vi "IMU_Read_STATUS.vi"(8 "error in (no error)":errorcluster caption="Fehler (Eingang, kein Fehler)", 10 "VISA resource name IN":refnum<visa-resource-name>, 11 "MultiWii Data Cluster 2":refnum<vi>) -> (0 "error out":errorcluster caption="Fehler (Ausgang)", 2 "VISA resource name OUT":refnum<visa-resource-name>, 5 "Sensors Present":u16[](array[numeric]))   [LabVIEW 2017]
uses:
  IMU_Data_Cluster.ctl
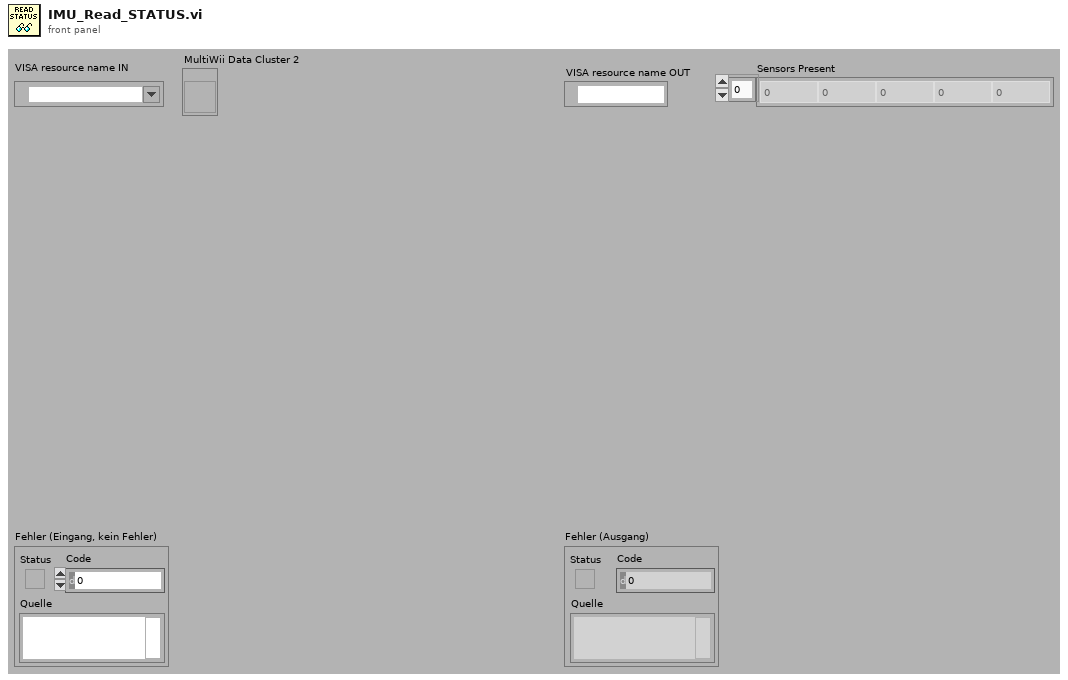
[diagram p1: front panel]
types:
  T1 = typedef "IMU_Data_Cluster.ctl" = cluster{"Firmware Revision":string, "Multitype Name":string, "Cycle Time":u16, "I²C Error Count":u16, "ACC present":bool, "Baro present":bool, "Mag Present":bool, "GPS present":bool, "Sonar present":bool, "Acc X axis (Roll)":dbl, "Acc Y axis (Pitch)":dbl, "Acc Z axis (Yaw)":dbl, "Gyro X axis (Roll)":dbl, "Gyro Y axis (Pitch)":dbl, "Gyro Z axis (Yaw)":dbl, "Mag X axis (Roll)":dbl, "Mag Y axis (Pitch)":dbl, "Mag Z axis (Yaw)":dbl, "X angle (Roll)":dbl, "Y angle (Pitch)":dbl, "Heading [°]":dbl, "Altitude [m]":dbl, "Vario":dbl, "GPS_Fix":u8, "GPS_NumSat":u8, "GPS_coord[LAT]":dbl, "GPS_coord[LON]":dbl, "GPS_Altitude":dbl, "GPS_Speed over Ground":dbl, "GPS_Ground Course":dbl, "Baro P [mbara]":dbl, "Baro T [°C]":dbl, "Altitude abs [m]":dbl}
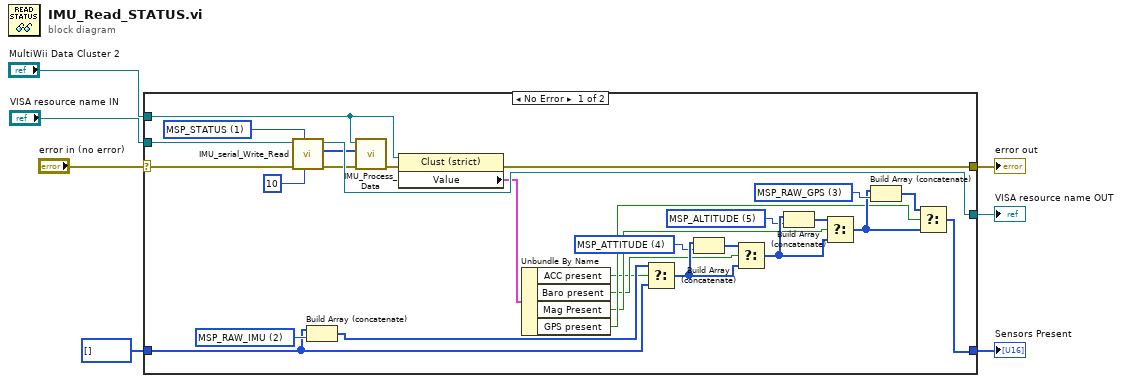
[diagram p0: block diagram]
diagram:
  n1 = case shown="No Error" "error in (no error)" {
    selector: "error in (no error)" -> [w14 w36]
    tunnel: "VISA resource name IN" -> [w35 w37]
    tunnel: [w34 w37] -> w6
    tunnel: [w8 w36] -> w5
    tunnel: [w15 w38] -> w4
    tunnel: u16[] [] -> [w13 w38]
    tunnel: "MultiWii Data Cluster 2" -> [w11 _]
    frame No Error {
      w22 = u16 3 items=["MSP_IDENT", "MSP_STATUS", "MSP_RAW_IMU", "MSP_RAW_GPS", "MSP_ATTITUDE", "MSP_ALTITUDE", "MSP_ACC_CALIBRATION", "MSP_MAG_CALIBRATION"] ("Command Selection")
      w28 = u16 5 items=["MSP_IDENT", "MSP_STATUS", "MSP_RAW_IMU", "MSP_RAW_GPS", "MSP_ATTITUDE", "MSP_ALTITUDE", "MSP_ACC_CALIBRATION", "MSP_MAG_CALIBRATION"] ("Command Selection")
      w25 = u16 4 items=["MSP_IDENT", "MSP_STATUS", "MSP_RAW_IMU", "MSP_RAW_GPS", "MSP_ATTITUDE", "MSP_ALTITUDE", "MSP_ACC_CALIBRATION", "MSP_MAG_CALIBRATION"] ("Command Selection")
      w23 = u16 2 items=["MSP_IDENT", "MSP_STATUS", "MSP_RAW_IMU", "MSP_RAW_GPS", "MSP_ATTITUDE", "MSP_ALTITUDE", "MSP_ACC_CALIBRATION", "MSP_MAG_CALIBRATION"] ("Command Selection")
      w31 = u16 1 items=["MSP_IDENT", "MSP_STATUS", "MSP_RAW_IMU", "MSP_RAW_GPS", "MSP_ATTITUDE", "MSP_ALTITUDE", "MSP_ACC_CALIBRATION", "MSP_MAG_CALIBRATION"] ("Command Selection")
      n2 = call "IMU_serial_Write_Read.vi"("Delay (ms)"=u32 10, "Command Selection"=w31, "error in (no error)"=w14, "VISA resource name IN"=w35) -> ("error IO"=w33:errorcluster, "Received Raw Data Byte-Array U8"=w32:u8[], "VISA resource name OUT"=w34:refnum<visa-resource-name>)  [unwired: 5 in]
      n3 = Build Array (concatenate)(w13, w23) -> (w24:u16[])
      n4 = call "IMU_Process_Data.vi"("error in (no error)"=w33, "Received Raw Data Byte-Array U8"=w32, "MultiWii Data Cluster 2"=w11) -> ("error out"=w9:errorcluster)  [unwired: 8 in]
      n5 = property class="Clust (strict)"(reference=w11, error in=w9) -> (error out=w8:errorcluster, "Value"=w10:T1)  [unwired: 1 out]
      n6 = Unbundle By Name(w10) -> ("ACC present"=w16:bool, "Baro present"=w17:bool, "Mag Present"=w18:bool, "GPS present"=w19:bool)
      n7 = Select(t=w24, s=w16, f=w13) -> (s? t:f=w26:u16[])
      n8 = Build Array (concatenate)(w26, w25) -> (w27:u16[])
      n9 = Select(t=w27, s=w17, f=w26) -> (s? t:f=w29:u16[])
      n10 = Build Array (concatenate)(w29, w28) -> (w30:u16[])
      n11 = Select(t=w30, s=w18, f=w29) -> (s? t:f=w20:u16[])
      n12 = Build Array (concatenate)(w20, w22) -> (w21:u16[])
      n13 = Select(t=w21, s=w19, f=w20) -> (s? t:f=w15:u16[])
    }
    frame Error {
    }
  }
  "VISA resource name OUT" <- w6
  "error out" <- w5
  "Sensors Present" <- w4
